vi "FTW-DevUtil-FindVIsWithSelectedFPItems.vi"() -> ()   [LabVIEW 2015]
panel:
  out "error out":errorcluster
  out "Array":path[](array[path])
  in  "Path":path
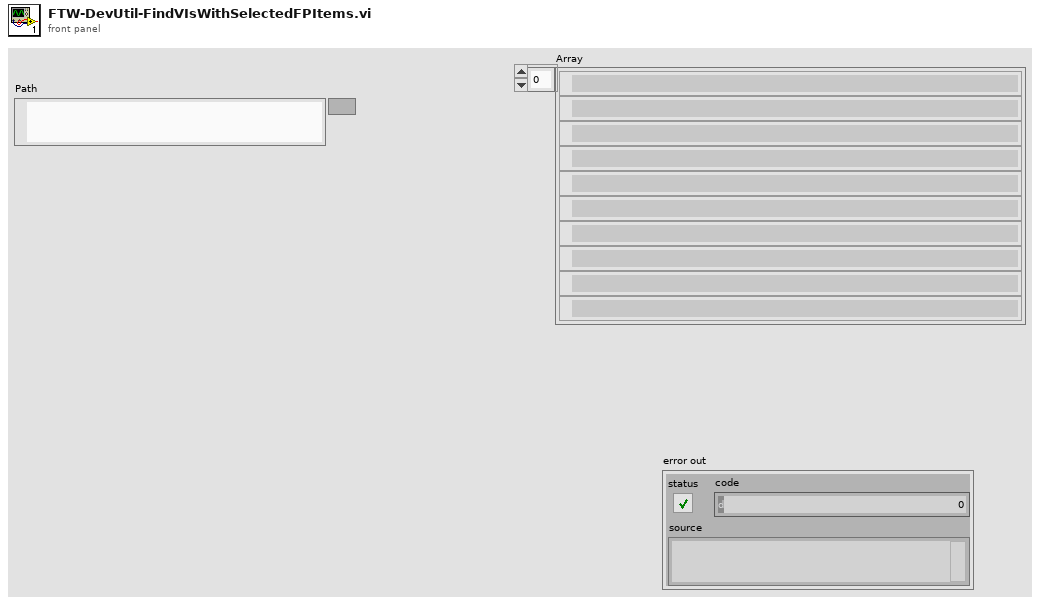
[diagram p1: front panel]
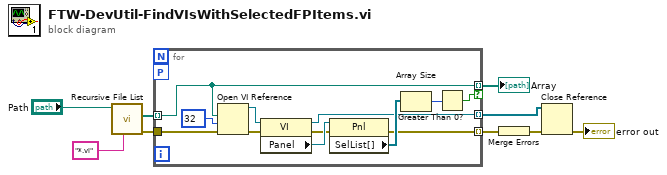
[diagram p0: block diagram]
diagram:
  n1 = call <vilib>:"Recursive File List.vi"("pattern"="*.vi", "Folder Path"="Path") -> ("error out"=w3:errorcluster, "All Files in Dir"=w7:path[])  [unwired: 5 in, 3 out]
  n2 = for {
    tunnel: w7 -> [w15] mode=indexing
    tunnel: [w15] -> w6 mode=indexing if=w13
    tunnel: [w12] -> w5 mode=indexing
    tunnel: w3 -> [w11]
    tunnel: [w10] -> w1 mode=indexing
    workers-P: _ -> [_]
    n3 = Open VI Reference(vi path=w15, options=32, error in (no error)=w11) -> (vi reference=w20:refnum<vi>, error out=w19:errorcluster)  [unwired: 3 in]
    n4 = property class="VI"(reference=w20, error in=w19) -> (reference out=w10:refnum<vi>, error out=w17:errorcluster, "Panel"=w18:refnum<vi>)
    n5 = property class="Pnl"(reference=w18, error in=w17) -> (error out=w12:errorcluster, "SelList[]"=w16:refnum<vi>[])  [unwired: 1 out]
    n6 = Array Size(array=w16) -> (size(s)=w14:i32)
    n7 = Greater Than 0?(x=w14) -> (x > 0?=w13:bool)
  }
  "Array" <- w6
  n8 = Merge Errors(w5) -> (w4:errorcluster)
  n9 = Close Reference(reference=w1, error in (no error)=w4) -> (error out=→"error out":errorcluster)
